vi "View Results.vi"(8 "error in (no error)":errorcluster, 11 "Results":T3=[{"Time Stamp"=timestamp(3677175403.0555263 s since 1904-01-01), "Port Number"=82, "Communication Type"=enum."TCP - Server to Client", "success?"=TRUE, "error in"={"status"=FALSE, "code"=0, "source"=""}}, {"Time Stamp"=timestamp(3677175404.082499 s since 1904-01-01), "Port Number"=482, "Communication Type"=enum."TCP - Server to Client", "success?"=TRUE, "error in"={"status"=FALSE, "code"=0, "source"=""}}, {"Time Stamp"=timestamp(3677175405.1130342 s since 1904-01-01), "Port Number"=5672, "Communication Type"=enum."TCP - Server to Client", "success?"=TRUE, "error in"={"status"=FALSE, "code"=0, "source"=""}}, {"Time Stamp"=timestamp(3677175406.136469 s since 1904-01-01), "Port Number"=6343, "Communication Type"=enum."TCP - Server to Client", "success?"=TRUE, "error in"={"status"=FALSE, "code"=0, "source"=""}}, {"Time Stamp"=timestamp(3677175407.1725154 s since 1904-01-01), "Port Number"=8002, "Communication Type"=enum."TCP - Server to Client", "success?"=TRUE, "error in"={"status"=FALSE, "code"=0, "source"=""}}, {"Time Stamp"=timestamp(3677175408.2013106 s since 1904-01-01), "Port Number"=49580, "Communication Type"=enum."TCP - Server to Client", "success?"=TRUE, "error in"={"status"=FALSE, "code"=0, "source"=""}}, {"Time Stamp"=timestamp(3677175409.236001 s since 1904-01-01), "Port Number"=3580, "Communication Type"=enum."TCP - Server to Client", "success?"=FALSE, "error in"={"status"=TRUE, "code"=56, "source"="TCP Read in Test Server to Client (TCP).vi->Main.vi"}}, {"Time Stamp"=timestamp(3677175411.2628417 s since 1904-01-01), "Port Number"=80, "Communication Type"=enum."TCP - Server to Client", "success?"=FALSE, "error in"={"status"=TRUE, "code"=56, "source"="TCP Read in Test Server to Client (TCP).vi->Main.vi"}}, {"Time Stamp"=timestamp(3677175413.268388 s since 1904-01-01), "Port Number"=22, "Communication Type"=enum."TCP - Server to Client", "success?"=TRUE, "error in"={"status"=FALSE, "code"=0, "source"=""}}, {"Time Stamp"=timestamp(3677175414.271773 s since 1904-01-01), "Port Number"=44516, "Communication Type"=enum."TCP - Server to Client", "success?"=TRUE, "error in"={"status"=FALSE, "code"=0, "source"=""}}, {"Time Stamp"=timestamp(3677175415.2839184 s since 1904-01-01), "Port Number"=52725, "Communication Type"=enum."TCP - Server to Client", "success?"=TRUE, "error in"={"status"=FALSE, "code"=0, "source"=""}}, {"Time Stamp"=timestamp(3677175416.31165 s since 1904-01-01), "Port Number"=8080, "Communication Type"=enum."TCP - Server to Client", "success?"=FALSE, "error in"={"status"=TRUE, "code"=56, "source"="TCP Read in Test Server to Client (TCP).vi->Main.vi"}}, {"Time Stamp"=timestamp(3677175418.324825 s since 1904-01-01), "Port Number"=5353, "Communication Type"=enum."UDP - Server to Client", "success?"=FALSE, "error in"={"status"=TRUE, "code"=60, "source"="UDP Open in UDP - Sender.vi->Main.vi"}}, {"Time Stamp"=timestamp(3677175420.333691 s since 1904-01-01), "Port Number"=44515, "Communication Type"=enum."UDP - Server to Client", "success?"=TRUE, "error in"={"status"=FALSE, "code"=0, "source"=""}}, {"Time Stamp"=timestamp(3677175421.33937 s since 1904-01-01), "Port Number"=44525, "Communication Type"=enum."UDP - Server to Client", "success?"=TRUE, "error in"={"status"=FALSE, "code"=0, "source"=""}}]) -> (0 "error out":errorcluster)   [LabVIEW 2019]
uses:
  controls/Results.ctl
  controls/Log Data Cluster.ctl
  controls/Communication Types.ctl
panel:
  in  "done":bool
  out "Results":T1[](array[typedef])
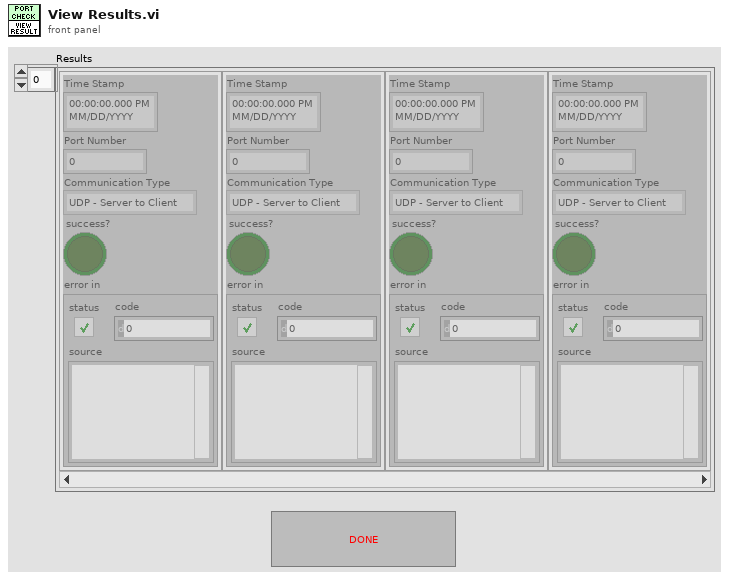
[diagram p1: front panel]
types:
  T1 = typedef "Log Data Cluster.ctl" = cluster{"Time Stamp":timestamp, "Port Number":u16, "Communication Type":T2, "success?":bool, "error in":errorcluster}
  T2 = typedef "Communication Types.ctl" = enum16{"UDP - Server to Client", "UDP - Client to Server", "TCP - Server to Client", "TCP - Client to Server"}
  T3 = typedef "Results.ctl" = T4[]
  T4 = typedef "log data cluster.ctl" = cluster{"Time Stamp":timestamp, "Port Number":u16, "Communication Type":T2, "success?":bool, "error in":errorcluster}
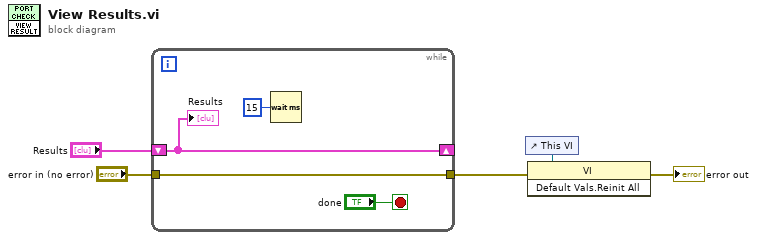
[diagram p0: block diagram]
diagram:
  n1 = while {
    shift-right: [w9] -> _
    shift-left: "Results" -> [w9]
    tunnel: [w6] -> w1
    tunnel: "error in (no error)" -> [w6]
    stop <- "done" stop-if-true
    n2 = Wait (ms)(milliseconds to wait=u32 15) -> ()  [unwired: 1 out]
    "Results" <- w9
  }
  n3 = control-ref of="This VI"() -> (w4:refnum<vi>)
  n4 = invoke class="VI" method="Default Vals.Reinit All"(reference=w4, error in=w1) -> (error out=→"error out":errorcluster)  [unwired: 1 in, 2 out]
